vi "XY Graph Plot Interpolation.vi"(8 "error in (no error)":errorcluster, 10 "Active Plot":u32, 11 "XYGraph in":T1) -> (0 "error out":errorcluster, 2 "Bin Location":T2, 3 "Plot Interpolation":u8)   [LabVIEW 2021, in "XY Graph Add-Ons.lvlib"]
doc: "Returns the type of plot (display) interpolation used in the <B>XY Graph</B>."
uses:
  XY Graph Add-Ons.lvlib
  Histograms/Histogram Bin Position.ctl
  XY Graph Refnum.ctl
  Histograms/Histogram Window.lvlib
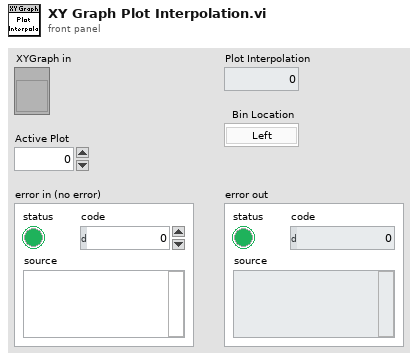
[diagram p1: front panel]
types:
  T1 = typedef "XY Graph Add-Ons.lvlib/XY Graph Refnum.ctl" = refnum<vi>
  T2 = typedef "Histogram Window.lvlib/Histogram Bin Position.ctl" = enum16{"Left", "Center", "Right"}
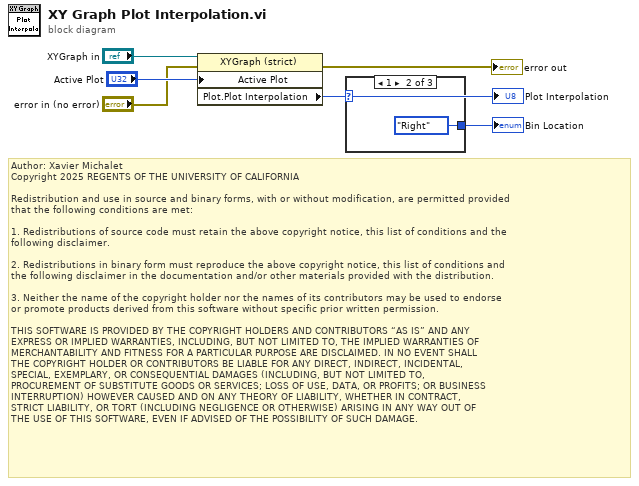
[diagram p0: block diagram]
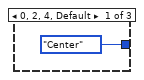
[diagram p2: hidden frame]
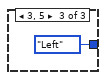
[diagram p3: hidden frame]
diagram:
  # "Author: Xavier Michalet\nCopyright 2025 REGENTS OF THE UNIVERSITY OF CALIFORNIA\n\nRedistribution and use in source and binary forms, with or without modification, are permitted provided\nthat the following conditions are met:\n\n1. Redistributions of source code must retain the above copyright notice, this list of conditions and the\nfollowing disclaimer.\n\n2. Redistributions in binary form must reproduce the above copyright notice, this list of conditions and\nthe following disclaimer in the documentation and/or other materials provided with the distribution.\n\n3. Neither the name of the copyright holder nor the names of its contributors may be used to endorse \nor promote products derived from this software without specific prior written permission.\n\nTHIS SOFTWARE IS PROVIDED BY THE COPYRIGHT HOLDERS AND CONTRIBUTORS “AS IS” AND ANY \nEXPRESS OR IMPLIED WARRANTIES, INCLUDING, BUT NOT LIMITED TO, THE IMPLIED WARRANTIES OF\nMERCHANTABILITY AND FITNESS FOR A PARTICULAR PURPOSE ARE DISCLAIMED. IN NO EVENT SHALL\nTHE COPYRIGHT HOLDER OR CONTRIBUTORS BE LIABLE FOR ANY DIRECT, INDIRECT, INCIDENTAL, \nSPECIAL, EXEMPLARY, OR CONSEQUENTIAL DAMAGES (INCLUDING, BUT NOT LIMITED TO, \nPROCUREMENT OF SUBSTITUTE GOODS OR SERVICES; LOSS OF USE, DATA, OR PROFITS; OR BUSINESS\nINTERRUPTION) HOWEVER CAUSED AND ON ANY THEORY OF LIABILITY, WHETHER IN CONTRACT, \nSTRICT LIABILITY, OR TORT (INCLUDING NEGLIGENCE OR OTHERWISE) ARISING IN ANY WAY OUT OF\nTHE USE OF THIS SOFTWARE, EVEN IF ADVISED OF THE POSSIBILITY OF SUCH DAMAGE."
  n1 = property class="XYGraph (strict)"(reference="XYGraph in", error in="error in (no error)", "Active Plot"="Active Plot") -> (error out=→"error out":errorcluster, "Plot.Plot Interpolation"=w5:u8)  [unwired: 1 out]
  "Plot Interpolation" <- w5
  n2 = case shown="1" w5 {
    tunnel: [Histogram_Bin_Position."Center" ("Bin Location") Histogram_Bin_Position."Right" ("Bin Location") Histogram_Bin_Position."Left" ("Bin Location")] -> w6
    frame 0, 2, 4, Default {
    }
    frame 1 {
    }
    frame 3, 5 {
    }
  }
  "Bin Location" <- w6
